vi "Create Control (to dir).vi"(8 "error in (no error)":errorcluster, 10 "Target Folder or .ctl":path, 11 "Control in":refnum<class "Control.lvclass">) -> (0 "error out":errorcluster, 3 "Control out":refnum<class "Control.lvclass">)   [LabVIEW 2013, in "uitools_Control.lvlib" / "Control.lvclass"]
uses:
  Control.lvclass
  <userlib>/_OpenG.lib/file/file.llb/Strip Path Extension - Path__ogtk.vi
  <userlib>/_OpenG.lib/file/file.llb/Strip Path - Arrays__ogtk.vi
  <userlib>/_OpenG.lib/file/file.llb/Build Path - Traditional__ogtk.vi
  <userlib>/BitMan/BitMap class/BitMap.lvclass
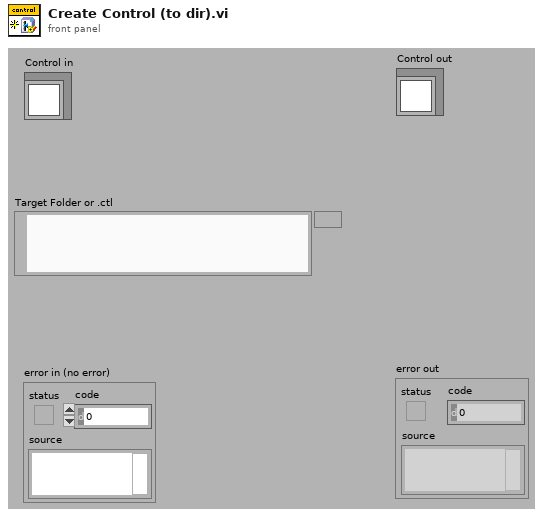
[diagram p1: front panel]
types:
  T1 = typedef "imagedata.ctl" = cluster{"image type":i32, "image depth":i32, "image":u8[], "mask":u8[], "colors":u32[], "Rectangle":cluster{"left":i16, "top":i16, "right":i16, "bottom":i16}}
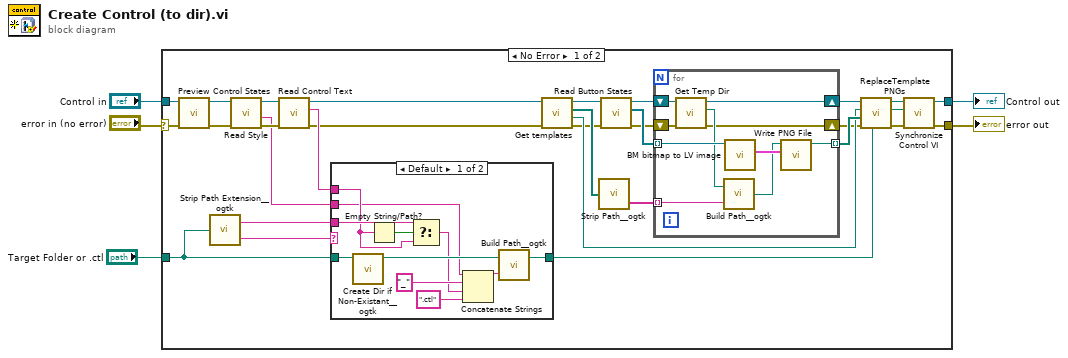
[diagram p0: block diagram]
diagram:
  n1 = case shown="No Error" "error in (no error)" {
    selector: "error in (no error)" -> [w17 w59]
    tunnel: [w23 w59] -> w2
    tunnel: [w24 w58] -> w3
    tunnel: "Control in" -> [w19 w58]
    tunnel: "Target Folder or .ctl" -> [w15 _]
    frame No Error {
      n2 = call-dynamic "Preview Control States.vi"("error in"=w17, "Control in"=w19) -> ("error out"=w16:errorcluster, "Control out"=w18:refnum<class "Control.lvclass">)  [unwired: 8 out]
      n3 = call-poly <userlib>:"Strip Path Extension__ogtk.vi"("path"=w15) -> ("root"=w14:string, "extension"=w6:string)
      n4 = call-dynamic "Read Style.vi"("error in (no error)"=w16, "Control in"=w18) -> ("error out"=w27:errorcluster, "Style name"=w13:string, "Control out"=w33:refnum<class "Control.lvclass">)  [unwired: 7 out]
      n5 = call-dynamic "Read Control Text.vi"("error in (no error)"=w27, "Control in"=w33) -> ("error out"=w9:errorcluster, "Control Text"=w11:string, "Control out"=w10:refnum<class "Control.lvclass">)  [unwired: 7 out]
      n6 = case shown="Default" w6 {
        tunnel: w15 -> [w46 w47]
        tunnel: w14 -> [w44 _]
        tunnel: w13 -> [w39 _]
        tunnel: [w37 w47] -> w12
        tunnel: w11 -> [w43 _]
        frame Default {
          n7 = call <userlib>:"Create Dir if Non-Existant__ogtk.vi"("Directory Path"=w46) -> ("dup Directory Path"=w40:path)  [unwired: 2 in, 8 out]
          n8 = Empty String/Path?(string/path=w43) -> (empty?=w45:bool)
          n9 = Select(t=w44, s=w45, f=w43) -> (s? t:f=w38:string)
          n10 = Concatenate Strings(w39, "_" ("string"), w38, ".ctl" ("string")) -> (w36:string)
          n11 = call-poly <userlib>:"Build Path__ogtk.vi"("name or relative path"=w36, "base path"=w40) -> ("appended path"=w37:path)
        }
        frame "ctl" {
        }
      }
      n12 = call-dynamic "Get templates.vi"("error in (no error)"=w9, "Control in"=w10) -> ("error out"=w25:errorcluster, "CTL template"=w32:path, "PNG templates"=w29:path[], "Control out"=w26:refnum<class "Control.lvclass">)  [unwired: 6 out]
      n13 = call-poly <userlib>:"Strip Path__ogtk.vi"("path"=w29) -> ("name"=w28:string[])  [unwired: 1 out]
      n14 = call-dynamic "Read Button States.vi"("error in (no error)"=w25, "Control in"=w26) -> ("error out"=w8:errorcluster, "Button States"=w35:refnum<class "BitMap.lvclass">[], "Control out"=w31:refnum<class "Control.lvclass">)  [unwired: 7 out]
      n15 = for {
        tunnel: [w55] -> w34 mode=indexing
        tunnel: w35 -> [w54] mode=indexing
        shift-right: [w52] -> w30
        shift-left: w31 -> [w53]
        tunnel: w28 -> [w50] mode=indexing
        shift-right: [w48] -> w7
        shift-left: w8 -> [w49]
        n16 = call-dynamic "Get Temp Dir.vi"("error in"=w49, "Control in"=w53) -> ("error out"=w48:errorcluster, "temp directory"=w51:path, "Control out"=w52:refnum<class "Control.lvclass">)  [unwired: 7 out]
        n17 = call-poly <userlib>:"Build Path__ogtk.vi"("name or relative path"=w50, "base path"=w51) -> ("appended path"=w56:path)
        n18 = call <userlib>:"BM bitmap to LV image.vi"("BitMap in"=w54) -> ("LV image data"=w57:T1)  [unwired: 2 in, 8 out]
        n19 = call <vilib>:"Write PNG File.vi"("image data"=w57, "path to PNG file"=w56) -> ("path"=w55:path)  [unwired: 1 in, 8 out]
      }
      n20 = call-dynamic "ReplaceTemplate PNGs.vi"("Control Destination"=w12, "error in"=w7, "States PNGs"=w34, "CTL template"=w32, "Control in"=w30) -> ("error out"=w21:errorcluster, "Control Destination dup"=w20:path, "Control out"=w22:refnum<class "Control.lvclass">)  [unwired: 4 out]
      n21 = call-dynamic "Synchronize Control VI.vi"("error in (no error)"=w21, "Control Destination"=w20, "Control in"=w22) -> ("error out"=w23:errorcluster, "Control out"=w24:refnum<class "Control.lvclass">)  [unwired: 7 out]
    }
    frame Error {
    }
  }
  "error out" <- w2
  "Control out" <- w3
